vi "Untitled 15 (SubVI).vi"(11 "Cluster":T3) -> (3 "Checkbox":bool)   [LabVIEW 2021]
uses:
  FW_producer_Data.ctl
  QMH_references_enum.ctl
  Framework_lib.lvlib
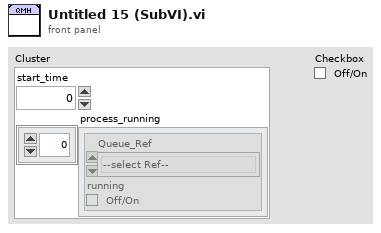
[diagram p1: front panel]
types:
  T1 = typedef "FW_producer_Data.ctl" = cluster{"Queue_Ref":T2, "running":bool}
  T2 = typedef "Framework_lib.lvlib/QMH_references_enum.ctl" = enum16{"--select Ref--", "Consumer_SUT", "Consumer_Annot", "Compute_Results"}
  T3 = cluster{"start_time":u32, "process_running":T1[]}
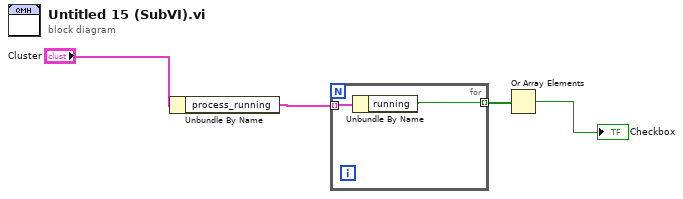
[diagram p0: block diagram]
diagram:
  n1 = Unbundle By Name("Cluster") -> ("process_running"=w2:T1[])
  n2 = for {
    tunnel: w2 -> [w6] mode=indexing
    tunnel: [w5] -> w3 mode=indexing
    n3 = Unbundle By Name(w6) -> ("running"=w5:bool)
  }
  n4 = Or Array Elements(Boolean array=w3) -> (logical OR=→"Checkbox":bool)
